vi "INIT.vi"(8 "error in (no error)":errorcluster, 11 "BD_PAPAS_USD_ES in":refnum<class "BD_PAPAS_USD_ES.lvclass">) -> (0 "error out":errorcluster, 3 "BD_PAPAS_USD_ES out":refnum<class "BD_PAPAS_USD_ES.lvclass">)   [LabVIEW 2019, in "BD_PAPAS_USD_ES.lvlib" / "BD_PAPAS_USD_ES.lvclass"]
uses:
  BD_PAPAS_USD_ES.lvclass
  BD_PAPAS_USD_ES.lvclass/BD_PAPAS_USD_ES.ctl
  Read MERCANCIA.vi
  Read VI Refnum.vi
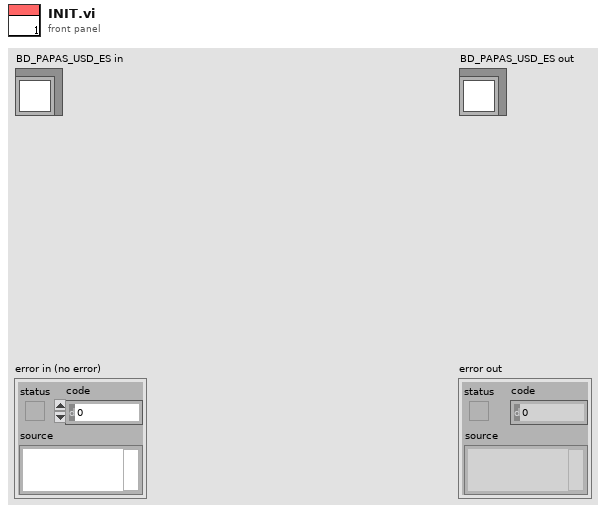
[diagram p1: front panel]
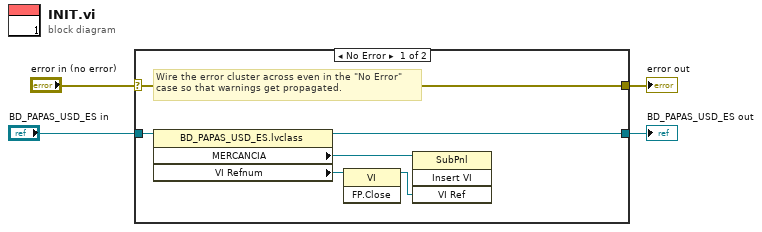
[diagram p0: block diagram]
diagram:
  n1 = case shown="No Error" "error in (no error)" {
    selector: "error in (no error)" -> [w9 w12]
    tunnel: [w9 w12] -> w3
    tunnel: [w8 w11] -> w1
    tunnel: "BD_PAPAS_USD_ES in" -> [w10 w11]
    frame No Error {
      # "Wire the error cluster across even in the \"No Error\"\ncase so that warnings get propagated."
      n2 = property class="BD_PAPAS_USD_ES.lvclass"(reference=w10) -> (reference out=w8:refnum<class "BD_PAPAS_USD_ES.lvclass">, "MERCANCIA"=w6:refnum<vi>, "VI Refnum"=w7:refnum<vi>)  [unwired: 1 in, 1 out]
      n3 = invoke class="VI" method="FP.Close"(reference=w7) -> (reference out=w5:refnum<vi>)  [unwired: 2 in, 2 out]
      n4 = invoke class="SubPnl" method="Insert VI"(reference=w6, "VI Ref"=w5) -> ()  [unwired: 2 in, 4 out]
    }
    frame Error {
    }
  }
  "error out" <- w3
  "BD_PAPAS_USD_ES out" <- w1
